vi "Write States.vi"(8 "error in (no error)":errorcluster, 10 "States":T1, 11 "AttackerBallOutOfFieldTactic in":refnum<class "AttackerBallOutOfFieldTactic.lvclass">) -> (0 "error out":errorcluster, 3 "AttackerBallOutOfFieldTactic out":refnum<class "AttackerBallOutOfFieldTactic.lvclass">)   [LabVIEW 2020, in "AttackerBallOutOfFieldTactic.lvclass"]
uses:
  AttackerBallOutOfFieldTactic.lvclass
  States.ctl
  AttackerBallOutOfFieldTactic.lvclass/AttackerBallOutOfFieldTactic.ctl
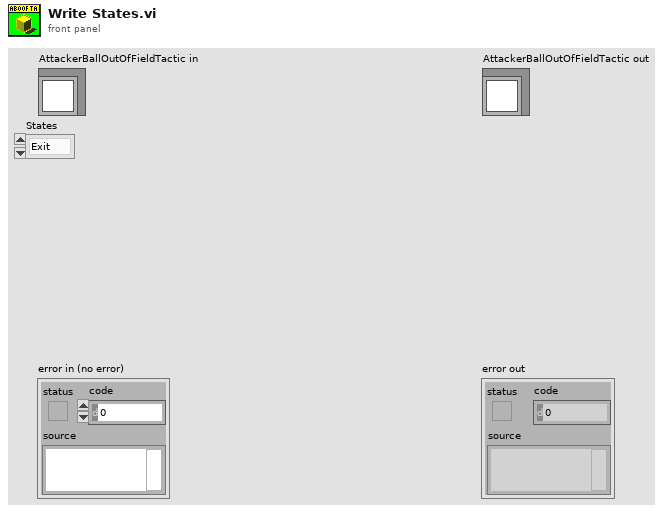
[diagram p1: front panel]
types:
  T1 = typedef "AttackerBallOutOfFieldTactic.lvclass/States.ctl" = enum16{"Exit", "BallOutOfField"}
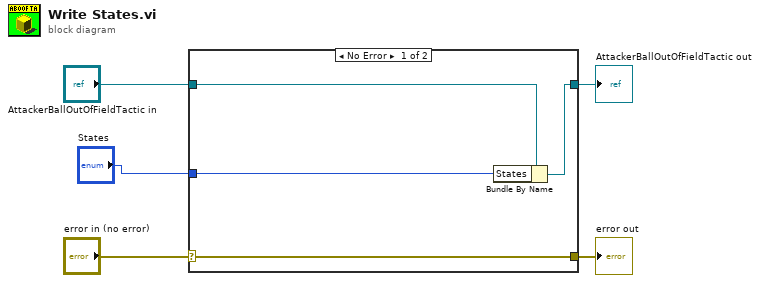
[diagram p0: block diagram]
diagram:
  n1 = case shown="No Error" "error in (no error)" {
    selector: "error in (no error)" -> [w9 w10]
    tunnel: [w9 w10] -> w4
    tunnel: [w7 w11] -> w2
    tunnel: "AttackerBallOutOfFieldTactic in" -> [w8 w11]
    tunnel: "States" -> [w6 _]
    frame No Error {
      n2 = Bundle By Name(cluster=w8, "States"=w6) -> (w7:refnum<class "AttackerBallOutOfFieldTactic.lvclass">)
    }
    frame Error {
    }
  }
  "error out" <- w4
  "AttackerBallOutOfFieldTactic out" <- w2
